vi "Get All Properties.vi"(8 "error in":errorcluster) -> (0 "error out":errorcluster, 3 "Properties[]":T1(array[cluster]))   [LabVIEW 2023]
panel:
  out "Classes processed":i32
  out "Class processing":string
  out "Property Ct":i32
  out "exe time (ms)":u32
  # "Original time was ca 5 min, improved class sorting and made sure we don't get properties for a class more than once:\n\n2504 props, 231 processed, 65s\n2504, 295 processed, 81s\n2504, 230 processed, 79s.\n\nLooks like sorting classes isn't needed\n\nNext round of improvement, put helper VI refs in shift registers so we don't get class and proeprty node rein a loop\n\n2504, props, 25s. Wow!!!\n\nLV2023 9-24\n2519 properties in 9.5s"
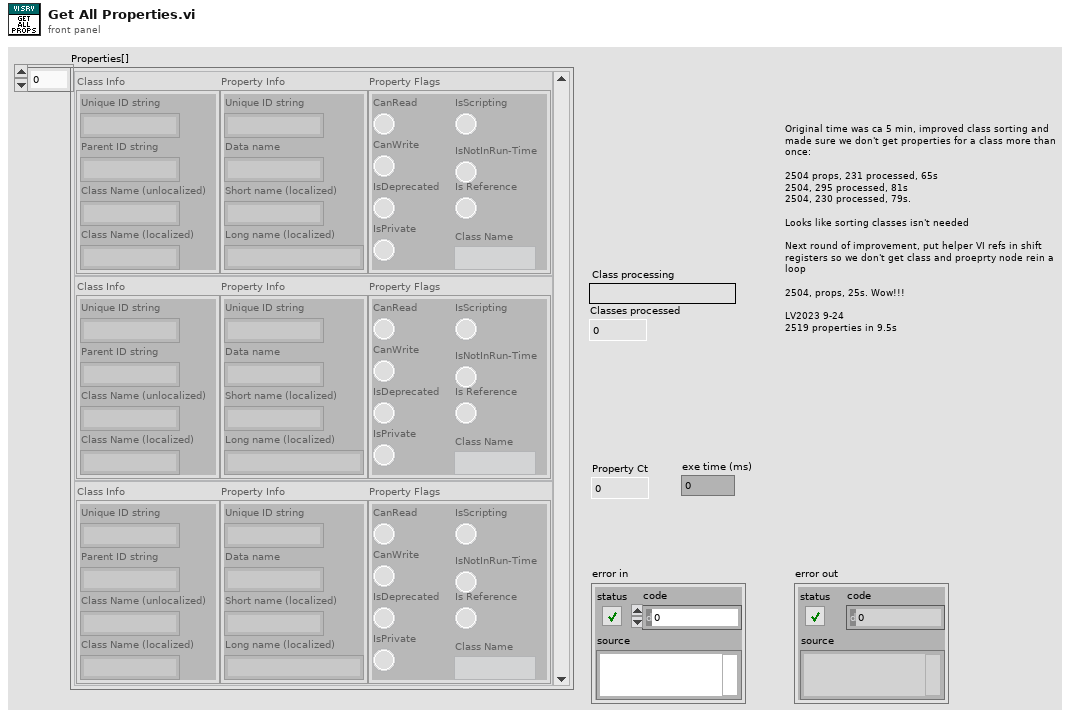
[diagram p1: front panel]
types:
  T1 = cluster{"Class Info":cluster{"Unique ID string":string, "Parent ID string":string, "Class Name (unlocalized)":string, "Class Name (localized)":string}, "Property Info":cluster{"Unique ID string":string, "Data name":string, "Short name (localized)":string, "Long name (localized)":string}, "Property Flags":cluster{"CanRead":bool, "CanWrite":bool, "IsDeprecated":bool, "IsPrivate":bool, "IsScripting":bool, "IsNotInRun-Time":bool, "Is Reference":bool, "Class Name":string}}[]
  T2 = cluster{"Unique ID string":string, "Parent ID string":string, "Class Name (unlocalized)":string, "Class Name (localized)":string}[]
  T3 = cluster{"Done":refnum<user-event>, "Msg 1":refnum<user-event>, "Msg 2":refnum<user-event>, "Prog Max":refnum<user-event>, "Prog Ct":refnum<user-event>}
  T4 = cluster{"Class Name":string, "Property Info":cluster{"Unique ID string":string, "Data name":string, "Short name (localized)":string, "Long name (localized)":string}}[]
  T5 = cluster{"Unique ID string":string, "Data name":string, "Short name (localized)":string, "Long name (localized)":string}
  T6 = cluster{"CanRead":bool, "CanWrite":bool, "IsDeprecated":bool, "IsPrivate":bool, "IsScripting":bool, "IsNotInRun-Time":bool, "Is Reference":bool, "Class Name":string}
  T7 = cluster{"Property/Method Info":cluster{"Unique ID string":string, "Parent ID string":string, "Class Name (unlocalized)":string, "Class Name (localized)":string}, "Property Info":cluster{"Unique ID string":string, "Data name":string, "Short name (localized)":string, "Long name (localized)":string}, "Property Flags":cluster{"CanRead":bool, "CanWrite":bool, "IsDeprecated":bool, "IsPrivate":bool, "IsScripting":bool, "IsNotInRun-Time":bool, "Is Reference":bool, "Class Name":string}}
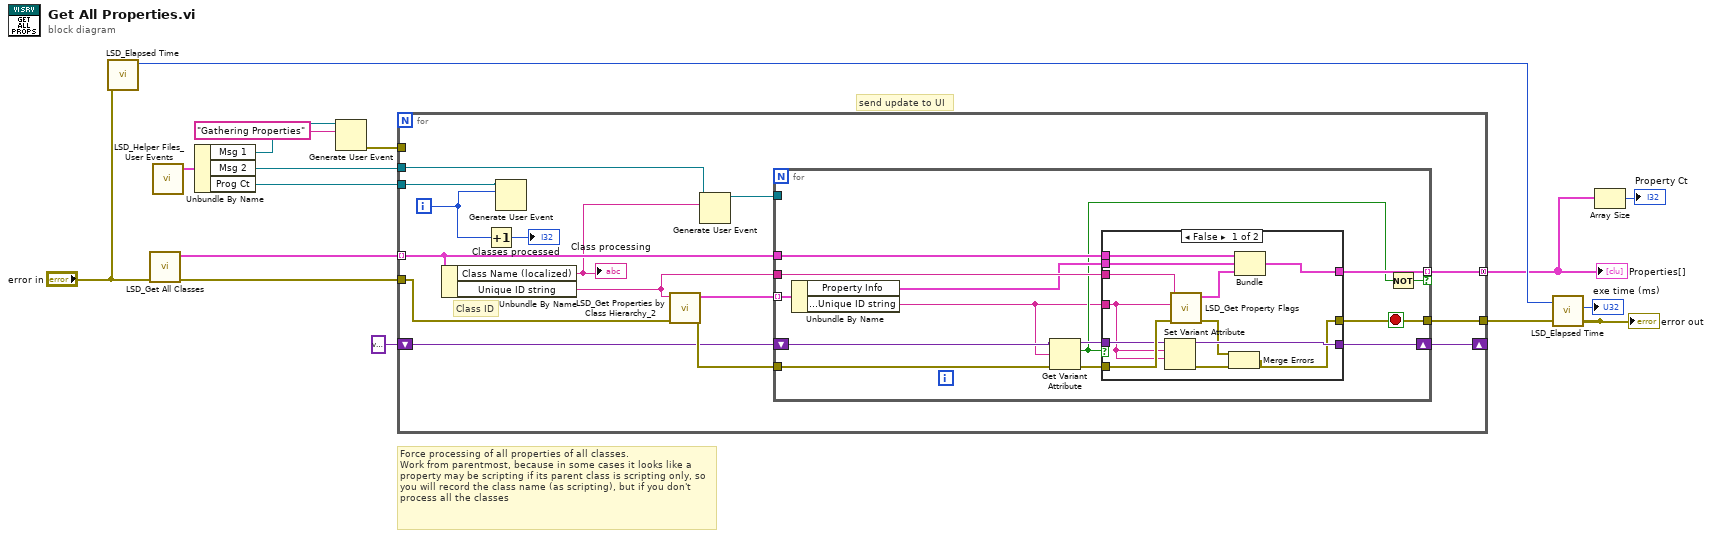
[diagram p0: block diagram]
diagram:
  # "send update to UI"
  # "Force processing of all properties of all classes.\nWork from parentmost, because in some cases it looks like a property may be scripting if its parent class is scripting only, so you will record the class name (as scripting), but if you don't process all the classes"
  n1 = call <resource>:"LSD_Elapsed Time.vi"("error in"="error in") -> ("millisecond timer value"=w13:u32)  [unwired: 6 in, 4 out]
  n2 = call <resource>:"LSD_Get All Classes.vi"("error in (no error)"="error in") -> ("error out"=w15:errorcluster, "VI Server Classes[]"=w10:T2)  [unwired: 9 in]
  n3 = call <resource>:"LSD_Helper Files_User Events.vi"() -> ("Init Dialog UEs"=w6:T3)  [unwired: 11 in]
  n4 = Unbundle By Name(w6) -> ("Msg 1"=w3:refnum<user-event>, "Msg 2"=w5:refnum<user-event>, "Prog Ct"=w4:refnum<user-event>)
  n5 = Generate User Event(user event=w3, event data cluster="Gathering Properties" ("event data")) -> (error out=w1:errorcluster)  [unwired: 2 in, 1 out]
  n6 = for {
    tunnel: w15 -> [w30]
    tunnel: [w22] -> w7
    shift-right: [w27] -> _
    shift-left: variant -> [w26]
    tunnel: [w24] -> w8 mode=concatenating
    tunnel: w10 -> [w21] mode=indexing
    tunnel: w5 -> [w20]
    tunnel: w4 -> [w18]
    tunnel: w1 -> [_]
    i -> [w17]
    # "Class ID"
    n7 = Unbundle By Name(w21) -> ("Class Name (localized)"=w16:string, "Unique ID string"=w25:string)
    "Class processing" <- w16
    n8 = Increment(x=w17) -> (x+1=→"Classes processed":i32)
    n9 = Generate User Event(user event=w18, event data cluster=w17) -> ()  [unwired: 2 in, 2 out]
    n10 = call <resource>:"LSD_Get Properties by Class Hierarchy_2.vi"("error in (no error)"=w30, "Class ID"=w25) -> ("error out"=w29:errorcluster, "Properties by Class Hierarchy"=w28:T4)  [unwired: 7 in, 1 out]
    n11 = Generate User Event(user event=w20, event data cluster=w16) -> (user event out=w19:refnum<user-event>)  [unwired: 2 in, 1 out]
    n12 = for {
      tunnel: w28 -> [w34] mode=indexing
      tunnel: w21 -> [w36]
      tunnel: w29 -> [w43]
      tunnel: [w44] -> w22
      shift-right: [w41] -> w27
      shift-left: w26 -> [w40]
      tunnel: w25 -> [w38]
      tunnel: [w37] -> w24 mode=indexing if=w32
      tunnel: w19 -> [_]
      stop <- w44 stop-if-true
      n13 = Unbundle By Name(w34) -> ("Property Info"=w35:T5, "Property Info.Unique ID string"=w31:string)
      n14 = Get Variant Attribute(Variant=w40, name=w31, error in=w43) -> (duplicate Variant=w39:variant, found=w33:bool, error out=w42:errorcluster)  [unwired: 1 in, 1 out]
      n15 = case shown="False" w33 {
        tunnel: w38 -> [w45 _]
        tunnel: w36 -> [w56 _]
        tunnel: [w46 w58] -> w44
        tunnel: w35 -> [w55 _]
        tunnel: w42 -> [w54 w58]
        tunnel: w31 -> [w49 _]
        tunnel: [w52 w57] -> w41
        tunnel: w39 -> [w51 w57]
        tunnel: [w50 _] -> w37
        frame False {
          n16 = Set Variant Attribute(Variant=w51, name=w49, value=w49) -> (Variant out=w52:variant, error out=w48:errorcluster)  [unwired: 1 in, 1 out]
          n17 = call <resource>:"LSD_Get Property Flags.vi"("error in (no error)"=w54, "Property ID"=w49, "Class ID"=w45) -> ("error out"=w47:errorcluster, "Property Flags"=w53:T6)  [unwired: 7 in]
          n18 = Merge Errors(w47, w48) -> (w46:errorcluster)
          n19 = Bundle("Property/Method Info"=w56, "Property Info"=w55, "Property Flags"=w53) -> (w50:T7)  [unwired: 1 in]
        }
        frame True {
        }
      }
      n20 = Not(x=w33) -> (.not. x?=w32:bool)
    }
  }
  "Properties[]" <- w8
  "error out" <- w7
  n21 = call <resource>:"LSD_Elapsed Time.vi"("error in"=w7, "past time"=w13) -> ("elapsed time (ms)"=→"exe time (ms)":u32)  [unwired: 5 in, 4 out]
  n22 = Array Size(array=w8) -> (size(s)=→"Property Ct":i32)
